vi "POS_R.vi"(8 "dt (s)":dbl=-1.0 caption="dt (초)" format="%.3f", 9 "Actual pos":i32, 10 "Pos_base_R":sgl) -> (0 "dt out (s)":dbl caption="dt 출력 (초)" format="%.3f", 3 "output":dbl caption="D_Vel" format="%.2f")   [LabVIEW 2019]
uses:
  <vilib>/addons/control/pid/pid.llb/PID (DBL).vi
  <vilib>/addons/control/pid/NI_PID_pid.lvlib
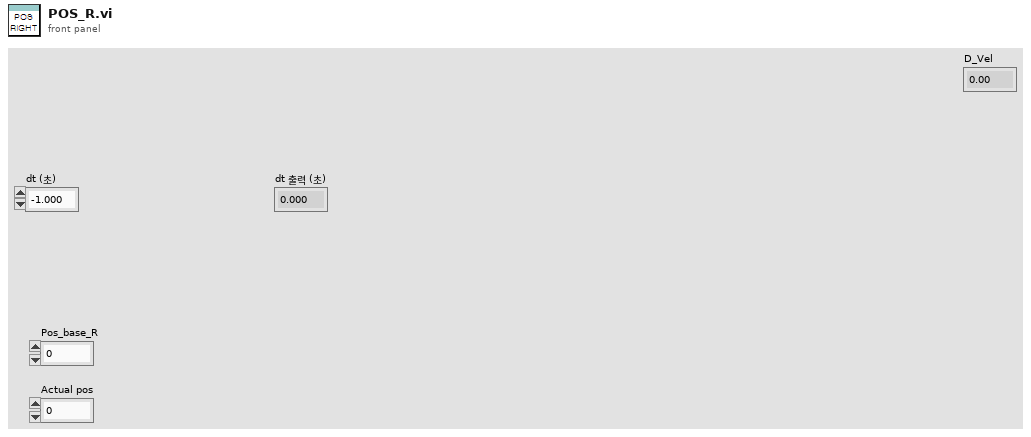
[diagram p1: front panel]
types:
  T1 = cluster{"proportional gain (Kc)":dbl, "integral time (Ti, min)":dbl, "derivative time (Td, min)":dbl}
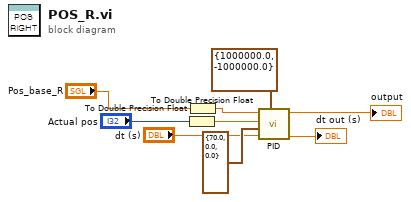
[diagram p0: block diagram]
diagram:
  n1 = To Double Precision Float(number="Actual pos") -> (double precision float=w2:dbl)
  n2 = To Double Precision Float(number="Pos_base_R") -> (double precision float=w3:dbl)
  n3 = call-poly <vilib>:"PID.vi"("output range"=cluster{"output high":dbl, "output low":dbl} {"output high"=1000000.0, "output low"=-1000000.0}, "dt (s)"="dt (s)", "PID gains"=T1 {"proportional gain (Kc)"=70.0, "integral time (Ti, min)"=0.0, "derivative time (Td, min)"=0.0}, "process variable"=w2, "setpoint"=w3) -> ("dt out (s)"=→"dt out (s)":dbl, "output"=→"output":dbl)  [unwired: 5 in]
